vi "自动搜索com口.vi"(0 "COM口列表输入":u16(ring) items=["COM1", "COM2"]) -> (1 "输出":refnum<visa-resource-name>, 2 "COM口列表输出":u16(ring) items=["COM1", "COM2"], 3 "查找列表":string[](array[string]), 4 "error IO":errorcluster)   [LabVIEW 2016]
uses:
  <vilib>/Instr/_visa.llb/VISA Find Search Mode.ctl
panel:
  out "序号":u16
  out "返回数":u32
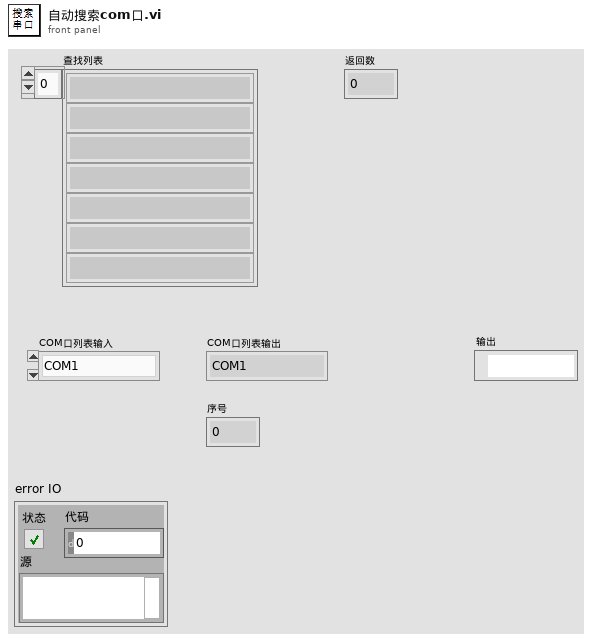
[diagram p1: front panel]
types:
  T1 = typedef "VISA Find Search Mode.ctl" = u32
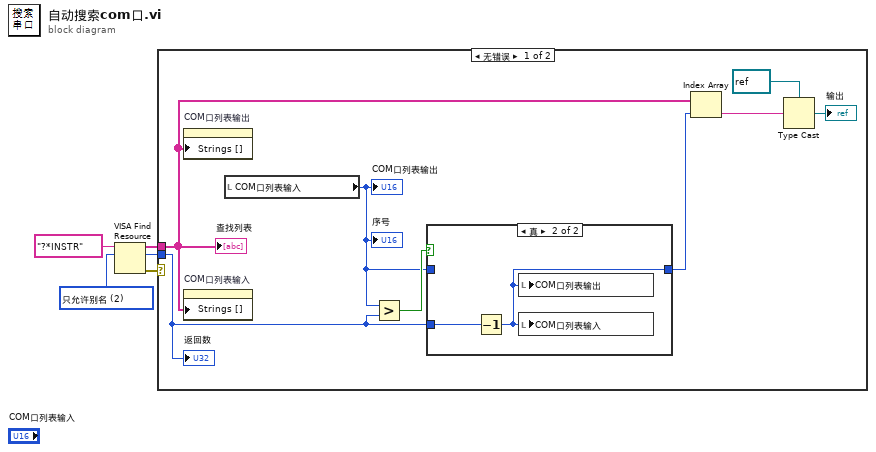
[diagram p0: block diagram]
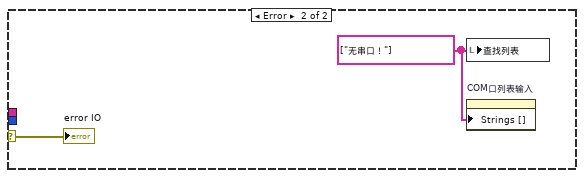
[diagram p3: hidden frame]
diagram:
  w4 = T1 2 items=["仅允许规范名称"=0, "只允许别名"=2, "包含匹配别名"=3, "包含所有别名"=4] ("Search Mode")
  n1 = VISA Find Resource(10:w4, 11:"?*INSTR" ("表达式(\"?*\")")) -> (0:w1:errorcluster, 2:w2:u32, 3:w3:string[])  [unwired: 1 in]
  n2 = case shown="无错误" w1 {
    selector: w1 -> [_ w17]
    tunnel: w3 -> [w7 _]
    tunnel: w2 -> [w13 _]
    frame No Error {
      n3 = property on="COM口列表输出" class="Ring (严格)"("Strings []"=w7) -> ()  [unwired: 2 in, 2 out]
      n4 = property on="COM口列表输入" class="Ring (严格)"("Strings []"=w7) -> ()  [unwired: 2 in, 2 out]
      n5 = local read "COM口列表输入"() -> (w8:u16)
      "序号" <- w8
      "COM口列表输出" <- w8
      n6 = Greater?(x=w8, y=w13) -> (0:w9:bool)
      n7 = case shown="真" w9 {
        tunnel: w13 -> [_ w16]
        tunnel: w8 -> [w14 _]
        tunnel: [w14 w15] -> w6
        frame False {
        }
        frame True {
          n8 = Decrement(x=w16) -> (x-1=w15:u32)
          n9 = local write "COM口列表输出"(w15) -> ()
          n10 = local write "COM口列表输入"(w15) -> ()
        }
      }
      n11 = Index Array(array=w7, index=w6) -> (element=w12:string)
      n12 = Type Cast(type=refnum<visa-resource-name> refnum ("VISA资源名称"), x=w12) -> (*(type *) &x=→"输出":refnum<visa-resource-name>)
      "返回数" <- w13
      "查找列表" <- w7
    }
    frame Error {
      w18 = string[] ["无串口！"] ("字符串[]")
      n13 = local write "查找列表"(w18) -> ()
      n14 = property on="COM口列表输入" class="Ring (严格)"("Strings []"=w18) -> ()  [unwired: 2 in, 2 out]
      "error IO" <- w17
    }
  }
